vi "Init EtherNet_IP Connection.vi"(2 "error in":errorcluster, 3 "EtherNet/IP Device Address":string="172.20.37.243") -> (0 "error out":errorcluster, 1 "Connection Cluster":T1={"TCP Connection"=refnum, "Session"=[], "EtherNet/IP Device Address"="172.20.37.243"} {"Session" format="0x%02x"})   [LabVIEW 2020, in "EtherNet_IP_Lib.lvlib"]
uses:
  EtherNet_IP_Lib.lvlib
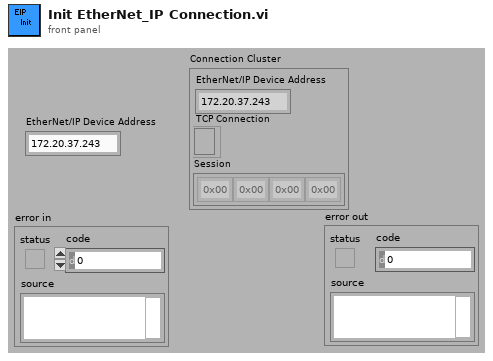
[diagram p1: front panel]
types:
  T1 = cluster{"TCP Connection":refnum<k5>, "Session":u8[], "EtherNet/IP Device Address":string}
  T2 = enum16{"Standard", "Buffered", "CRLF", "Immediate"}
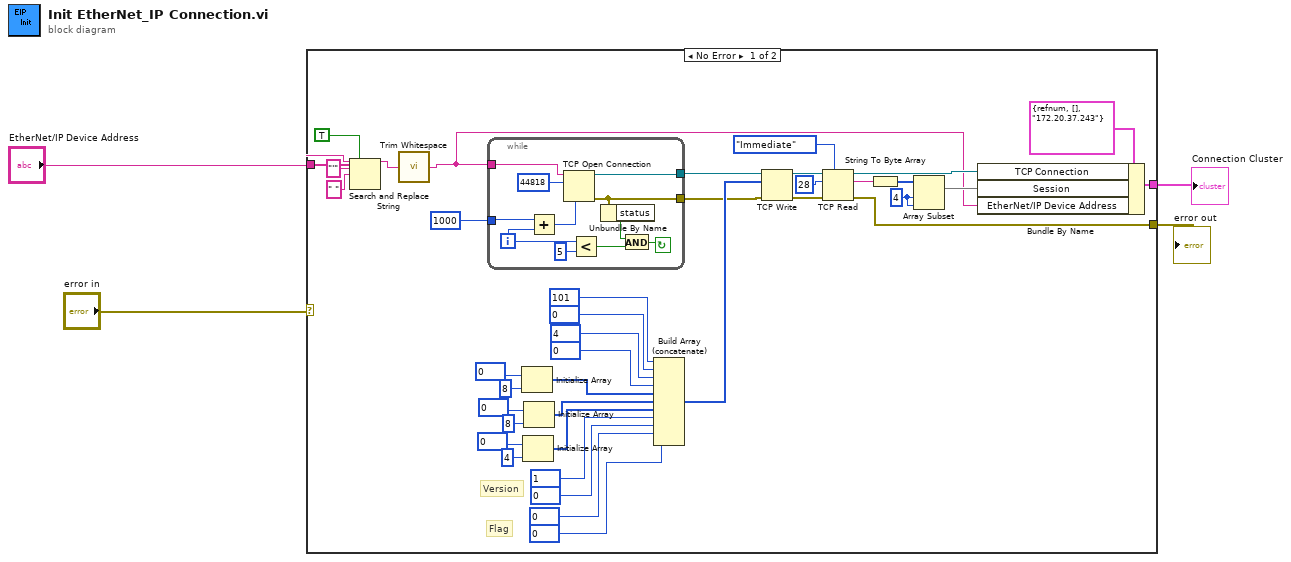
[diagram p0: block diagram]
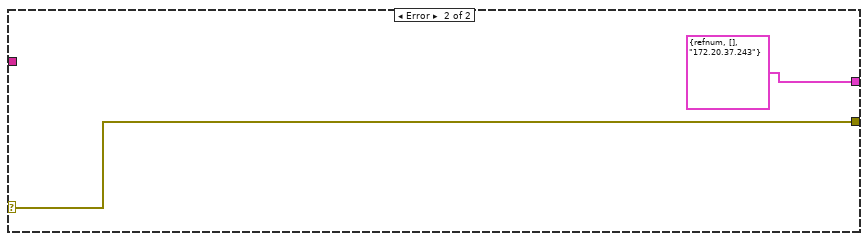
[diagram p2: hidden frame]
diagram:
  n1 = case shown="No Error" "error in" {
    selector: "error in" -> [_ w56]
    tunnel: "EtherNet/IP Device Address" -> [w9 _]
    tunnel: [w14 w56] -> w2
    tunnel: [w13 T1 {"TCP Connection"=refnum, "Session"=[], "EtherNet/IP Device Address"="172.20.37.243"} ("Connection Cluster")] -> w3
    frame No Error {
      w15 = 4 ("index")
      # "Flag"
      # "Version"
      n2 = Search and Replace String(replace all?=TRUE ("replace all? (F)"), input string=w9, search string="'", replace string=" " ("replace string (\"\")")) -> (result string=w8:string)  [unwired: 4 in, 3 out]
      n3 = call <vilib>:"Trim Whitespace.vi"("string"=w8) -> ("trimmed string"=w7:string)  [unwired: 1 in]
      n4 = while {
        tunnel: w7 -> [w54]
        tunnel: 1000 -> [w53]
        tunnel: [w50] -> w25
        tunnel: [w49] -> w21
        i -> [w48]
        stop <- w46 continue-if-true
        n5 = Add(x=w53, y=w48) -> (x+y=w51:i32)
        n6 = TCP Open Connection(address=w54, remote port or service name=u16 44818 ("remote port"), local port=w51) -> (connection ID=w50:refnum<k5>, error out=w49:errorcluster)  [unwired: 2 in]
        n7 = Less?(x=w48, y=5) -> (x < y?=w44:bool)
        n8 = Unbundle By Name(w49) -> ("status"=w45:bool)
        n9 = And(x=w45, y=w44) -> (x .and. y?=w46:bool)
      }
      n10 = Initialize Array(u8 0 ("Status"), 8 ("dimension size")) -> (w40:u8[])
      n11 = Initialize Array(u8 0 ("Status"), 4 ("dimension size")) -> (w26:u8[])
      n12 = Initialize Array(u8 0 ("Status"), 8 ("dimension size")) -> (w27:u8[])
      n13 = Build Array (concatenate)(u8 101 ("Status"), u8 0 ("Status"), u8 4 ("Status"), u8 0 ("Status"), w40, w27, w26, u8 1 ("Status"), u8 0 ("Status"), u8 0 ("Status"), u8 0 ("Status")) -> (w24:u8[])
      n14 = TCP Write(connection ID=w25, data in=w24, error in (no error)=w21) -> (connection ID out=w22:refnum<k5>, error out=w23:errorcluster)  [unwired: 1 in, 1 out]
      n15 = TCP Read(connection ID=w22, bytes to read=28, error in (no error)=w23, 7:T2."Immediate" ("mode (standard)")) -> (connection ID out=w19:refnum<k5>, data out=w18:string, error out=w14:errorcluster)  [unwired: 1 in]
      n16 = String To Byte Array(string=w18) -> (unsigned byte array=w17:u8[])
      n17 = Array Subset(array=w17, index=w15, length=w15) -> (w16:u8[])
      n18 = Bundle By Name(cluster=T1 {"TCP Connection"=refnum, "Session"=[], "EtherNet/IP Device Address"="172.20.37.243"} ("Connection Cluster"), "TCP Connection"=w19, "Session"=w16, "EtherNet/IP Device Address"=w7) -> (w13:T1)
    }
    frame Error {
    }
  }
  "Connection Cluster" <- w3
  "error out" <- w2
